vi "Play Song.vi"(0 "reference in":refnum<class "MusicPlayer.lvclass">, 11 "Error In":errorcluster) -> (4 "reference out":refnum<class "MusicPlayer.lvclass">, 15 "Error Out":errorcluster)   [LabVIEW 2022 SP3, in "MusicPlayer.lvclass"]
uses:
  MusicPlayer.lvclass
  MusicPlayer.lvclass/MusicPlayer.ctl
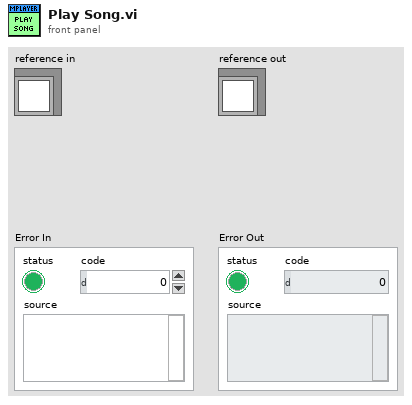
[diagram p1: front panel]
types:
  T1 = typedef "MusicPlayer.lvclass/ObjectAttributes.ctl" = cluster{"MediaPlayer":refnum<k7>, "Playlist":path[], "Index":u32}
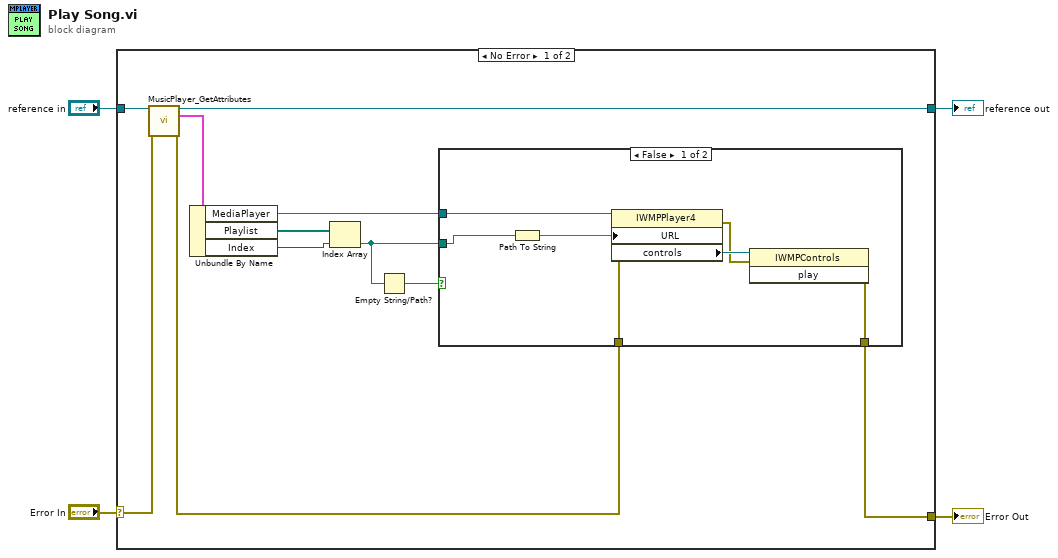
[diagram p0: block diagram]
diagram:
  n1 = case shown="No Error" "Error In" {
    selector: "Error In" -> [w15 w25]
    tunnel: [w10 w25] -> w3
    tunnel: [w12 w24] -> w1
    tunnel: "reference in" -> [w13 w24]
    frame No Error {
      n2 = call "MusicPlayer_GetAttributes.vi"("reference in"=w13, "error in (no error)"=w15) -> ("reference out"=w12:refnum<class "MusicPlayer.lvclass">, "Data"=w14:T1, "error out"=w9:errorcluster)  [unwired: 10 in, 1 out]
      n3 = Unbundle By Name(w14) -> ("MediaPlayer"=w11:refnum<k7>, "Playlist"=w8:path[], "Index"=w7:u32)
      n4 = Index Array(array=w8, index=w7) -> (element=w5:path)
      n5 = Empty String/Path?(string/path=w5) -> (empty?=w6:bool)
      n6 = case shown="False" w6 {
        tunnel: w11 -> [w22 _]
        tunnel: [w19 w23] -> w10
        tunnel: w9 -> [w18 w23]
        tunnel: w5 -> [w17 _]
        frame False {
          n7 = Path To String(path=w17) -> (string=w16:string)
          n8 = property class="IWMPPlayer4"(reference=w22, error in=w18, "URL"=w16) -> (error out=w20:errorcluster, "controls"=w21:refnum<k7>)  [unwired: 1 out]
          n9 = invoke class="IWMPControls" method="play"(reference=w21, error in=w20) -> (error out=w19:errorcluster)  [unwired: 1 in, 2 out]
        }
        frame True {
        }
      }
    }
    frame Error {
    }
  }
  "Error Out" <- w3
  "reference out" <- w1
